vi "CPP_CalcTubingCorrection.vi"() -> (5 "Plug in titles":string[](array[string]), 7 "Plug in values":string[](array[string]))   [LabVIEW 2020]
uses:
  <vilib>/Analysis/baseanly.llb/Mean (DBL).vi
  Globals/Meas_global.vi
  <vilib>/Analysis/NI_AALBase.lvlib
  <vilib>/Analysis/NI_AALPro.lvlib
panel:
  in  "Tab Control":enum32{"TubingCorrection", "Setup"}(tab)
  in  "RefXducer":i32(ring) items=["RV (Ref)", "RV (1)", "RV (2)", "RV (3)", "RV (4)", "RV (5)", "RV (6)", "RV (7)", "RV (8)", "RV (9)", "RV (10)", "RV (11)", "RV (12)", "RV (13)", "RV (14)", "RV (15)", "RV (16)", "RV (17)", "RV (18)", "RV (19)", "RV (20)", "RV (21)", "RV (22)", "RV (23)", "RV (24)", "RV (25)", "RV (26)", "RV (27)", "RV (28)", "RV (29)", "RV (30)", "RV (31)", "RV (32)", "RV (33)", "RV (34)", "RV (35)", "RV (36)", "RV (37)", "RV (38)", "RV (39)", "RV (40)", "RV (41)", "RV (42)", "RV (43)", "RV (44)", "RV (45)", "RV (46)", "RV (47)", "RV (48)", "RV (49)", "RV (50)", "RV (51)", "RV (52)", "RV (53)", "RV (54)", "RV (55)", "RV (56)", "RV (57)", "RV (58)", "RV (59)", "RV (60)", "RV (61)", "RV (62)", "RV (63)", "RV (64)"]
  in  "TestXducer":i32(ring) items=["RV (Ref)", "RV (1)", "RV (2)", "RV (3)", "RV (4)", "RV (5)", "RV (6)", "RV (7)", "RV (8)", "RV (9)", "RV (10)", "RV (11)", "RV (12)", "RV (13)", "RV (14)", "RV (15)", "RV (16)", "RV (17)", "RV (18)", "RV (19)", "RV (20)", "RV (21)", "RV (22)", "RV (23)", "RV (24)", "RV (25)", "RV (26)", "RV (27)", "RV (28)", "RV (29)", "RV (30)", "RV (31)", "RV (32)", "RV (33)", "RV (34)", "RV (35)", "RV (36)", "RV (37)", "RV (38)", "RV (39)", "RV (40)", "RV (41)", "RV (42)", "RV (43)", "RV (44)", "RV (45)", "RV (46)", "RV (47)", "RV (48)", "RV (49)", "RV (50)", "RV (51)", "RV (52)", "RV (53)", "RV (54)", "RV (55)", "RV (56)", "RV (57)", "RV (58)", "RV (59)", "RV (60)", "RV (61)", "RV (62)", "RV (63)", "RV (64)"]
  out "Time Traces":cluster{dbl, dbl, dbl[][]}(graph)
  out "Spectra":cluster{dbl, "df (Hz)":dbl, dbl[][]}(graph)
  in  "stop":bool
  in  "Pause Button":bool
  in  "Pause(ms)":u32=500
  in  "Coherence Threshold":dbl=0.98
  out "Coefficients Smoothed and Normalized":bool
  in  "Decimate Correction File?":bool=TRUE
  in  "Smooth Correction File?":bool=TRUE
  in  "CorrectionFileDestinationPath":path
  in  "fcut (Hz)":dbl=1000.0
  in  "Cutoff type":string(combo)="Brickwall"
  out "SD(boosted)":dbl format="%.3e"
  out "SD(ref)":dbl format="%.3e"
  out "SD(Boostederror%)":dbl format="%#_3g"
  out "Current Block No":i32
  in  "LowFrequencySmoothingFloor":dbl
  in  "LowFrequencySmoothingCeiling":dbl
  in  "ExistingTubingCorrectionFile":path
  in  "Apply Phase Correction?":bool=TRUE
  in  "Save Files?":bool
  in  "Use Existing Correction File?":bool
  out "df (Hz)":dbl format="%.6f"
  in  "Decimation Term":i32=10
  out "OutputString":string
  in  "N Points To Average Either Side":i32=10
  in  "Force Phase 0 Intercept?":bool=TRUE
  out "SD(muted)":dbl format="%.3e"
  out "SD(Mutederror%)":dbl format="%#_3g"
  # "#ToDo Must improve bottom end smoothing- DO NOT clamp to 1.00!!"
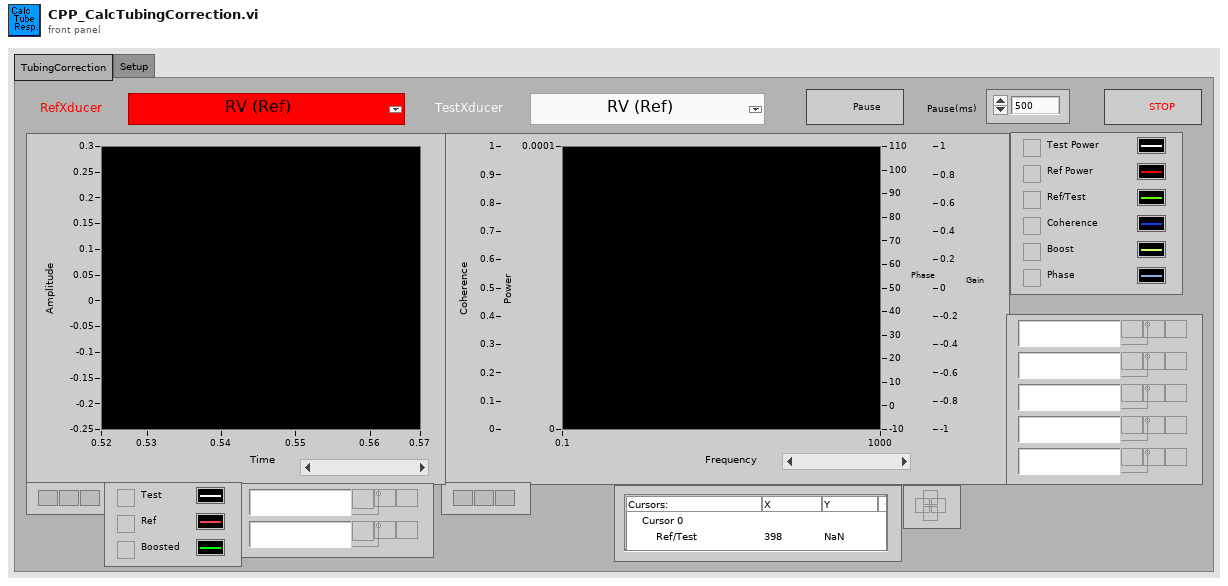
[diagram p1: front panel]
types:
  T1 = typedef "Analysis_info_cluster.ctl" = cluster{"Colour":u32, "Inst type":T2, "Inst name":string, "Symbol":string, "Code name":string, "Extra Info":string, "Inst Array":T3, "Extra Titles":string[], "Extra Values":string[], "U":dbl, "u^2":dbl, "u^3":dbl, "u^4":dbl, "Skew_u":dbl, "Kurt_u":dbl, "Sd Error in Mean":dbl, "% u'/U":dbl, "X":dbl, "Y":dbl, "Z":dbl, "Timescale integral Estimate":dbl, "Sd Error in Variance":dbl, "Calib File":path, "Calib Constants":dbl[], "Output Position":bool, "Stats":enum16{"None", "Basic", "Full"}, "Av Sampling Rate":dbl, "Av No of Samples":dbl, "Total Meas Time (s)":dbl, "ADAM Ch Name":string, "Max value":dbl, "Min value":dbl, "Req Sample Rate Hz":dbl, "Sync Delay Time (s)":dbl, "Ch No":i16, "Device":string, "Use Latest Calib":bool, "Port":string, "Metadata Ch Names":string[], "Metadata Ch Values":string[], "Label":string}
  T2 = typedef "Inst_type.ctl" = enum16{"Raw voltage", "Raw with zero offsetting", "Propeller anemometer", "Pressure Transducer", "Pitot-static tube", "Hot wire", "Cross wire 1", "Cross wire 2", "Generic Linear", "Generic Polynomial", "Generic BackPoly", "Fast FID", "Thermocouple", "Cold wire", "Pulsed Wire", "LDA Vel", "LDA Tran time", "LDA Arr time", "Microphone"}
  T3 = typedef "Instrument_Array.ctl" = enum16{"PWA", "LDA", "Analogue"}
  T4 = typedef "Time_Trace_Cluster.ctl" = cluster{"Weighting":dbl[], "Time (s)":dbl[], "Voltage":dbl[], "Eng Values":dbl[]}
  T5 = enum16{"open", "replace", "create", "open or create", "replace or create", "replace or create with confirmation"}
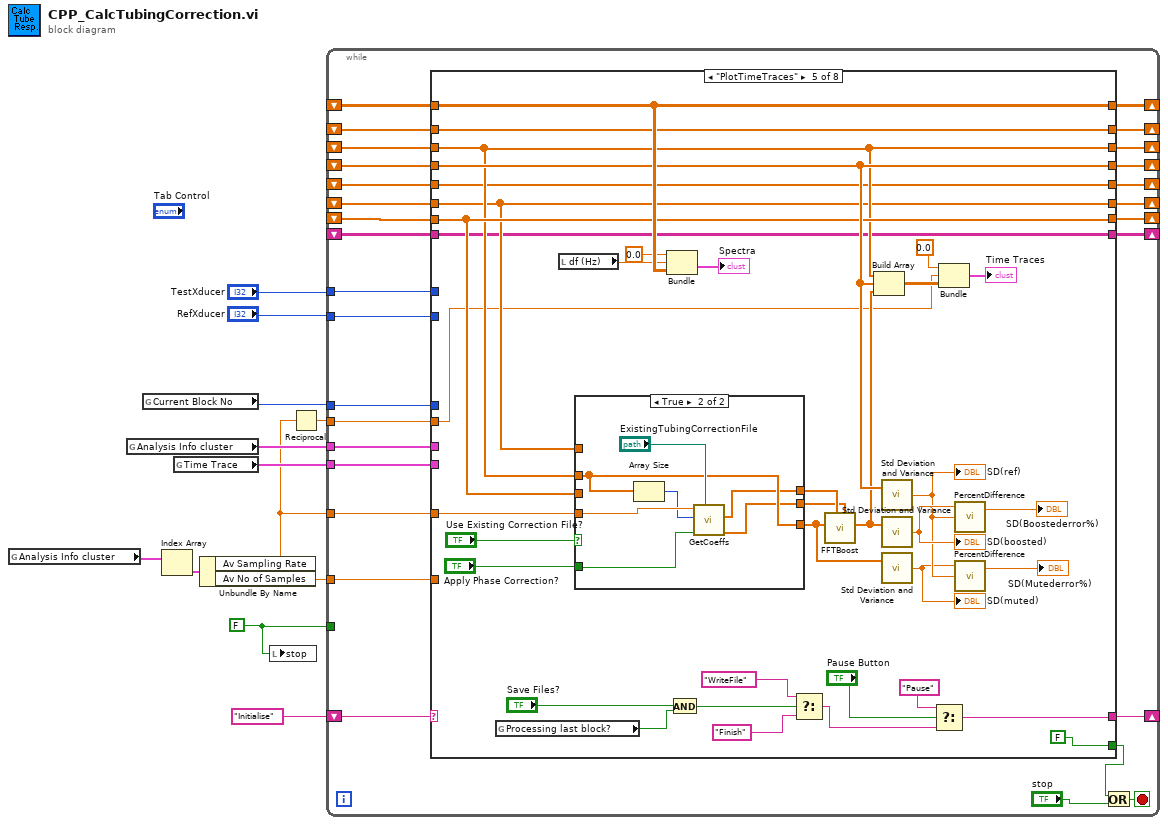
[diagram p0: block diagram]
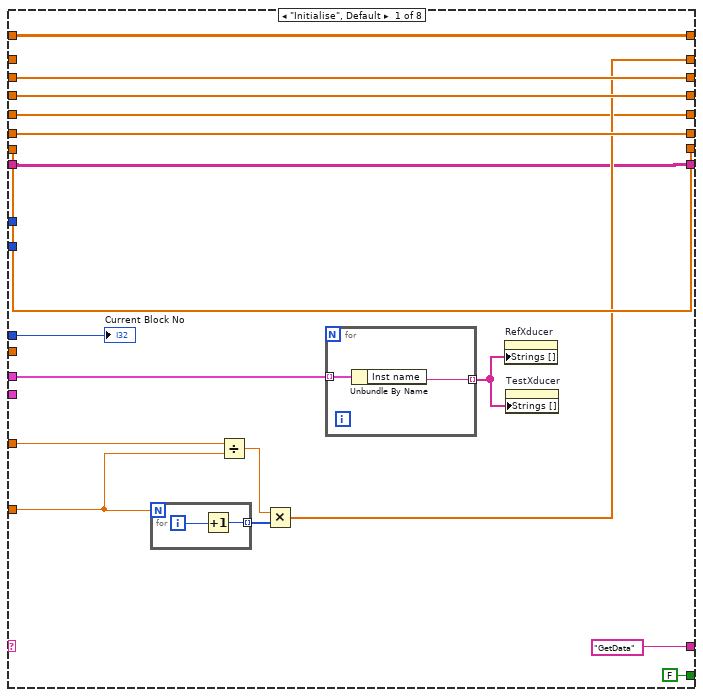
[diagram p2: hidden frame]
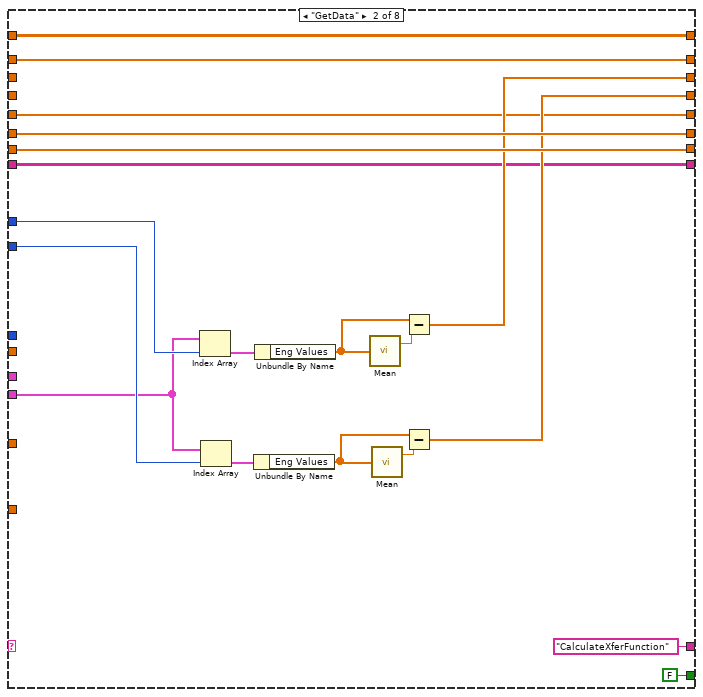
[diagram p3: hidden frame]
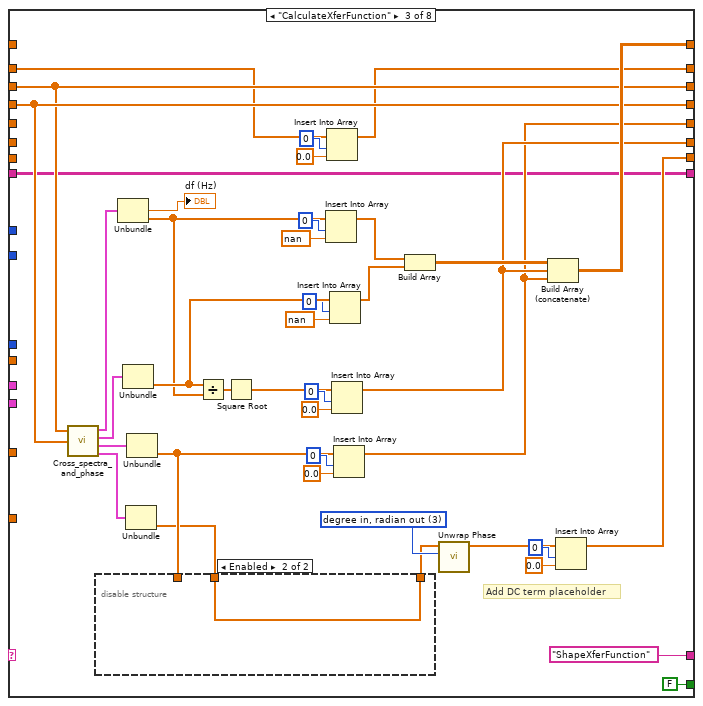
[diagram p4: hidden frame]
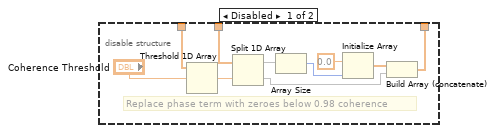
[diagram p5: hidden frame]
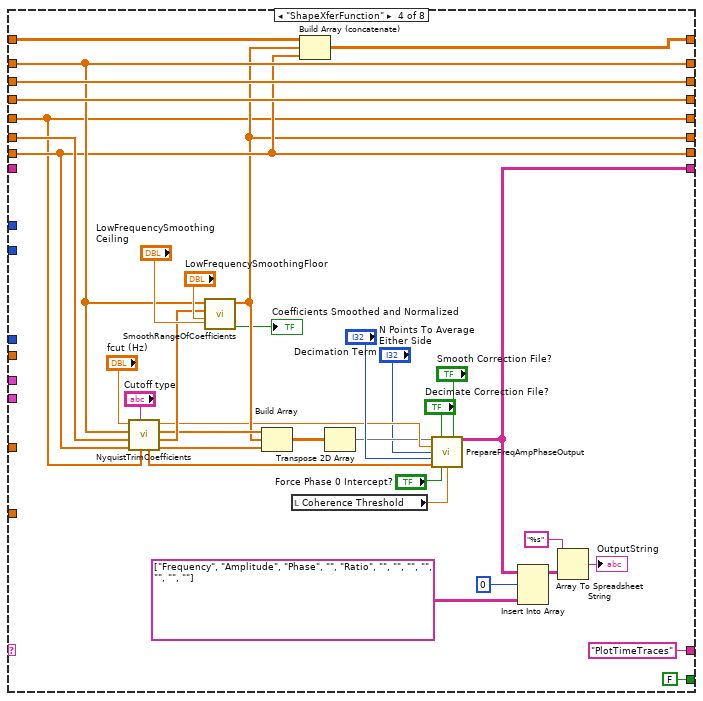
[diagram p6: hidden frame]
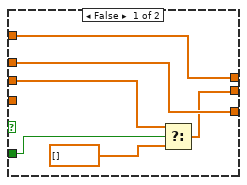
[diagram p7: hidden frame]
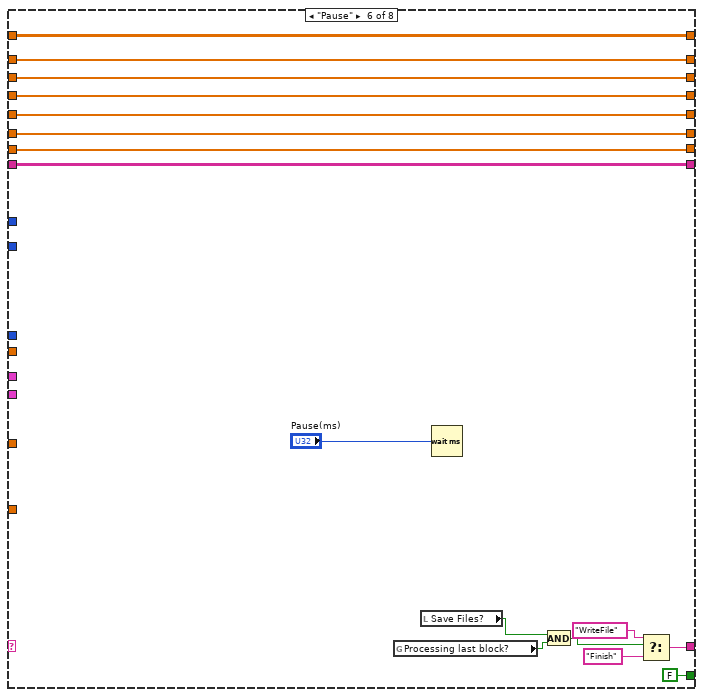
[diagram p8: hidden frame]
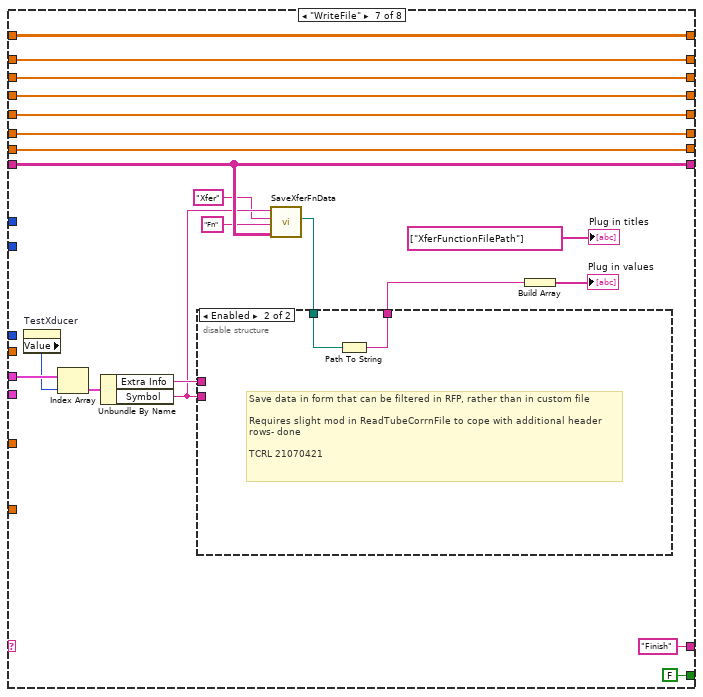
[diagram p9: hidden frame]
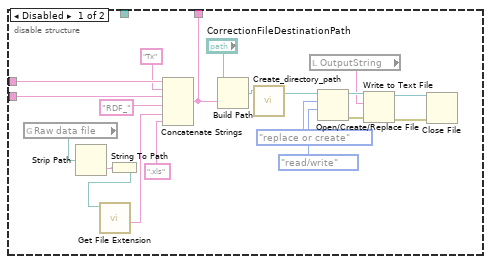
[diagram p10: hidden frame]
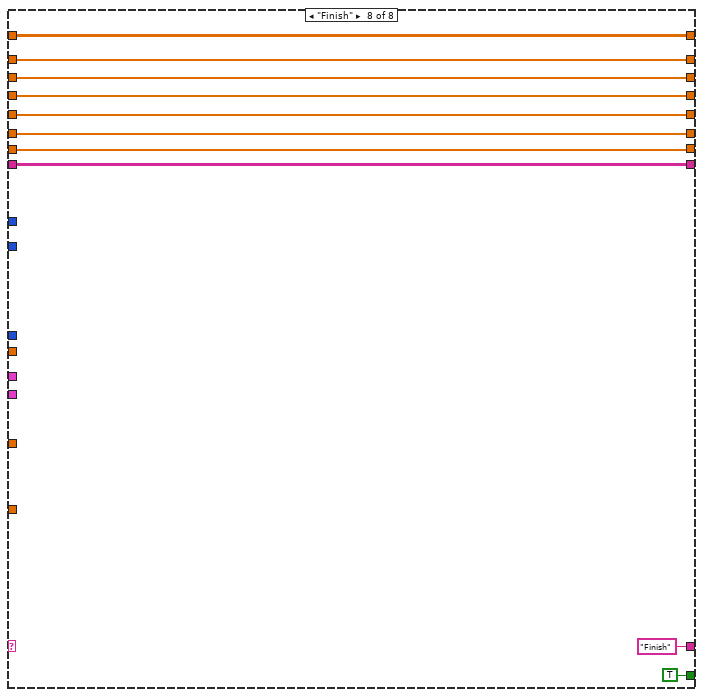
[diagram p11: hidden frame]
diagram:
  w11 = FALSE ("stop")
  n1 = global read "Meas_global.vi" "Analysis Info cluster"() -> (w5:T1[])
  n2 = global read "Meas_global.vi" "Analysis Info cluster"() -> (w8:T1[])
  n3 = global read "Meas_global.vi" "Current Block No"() -> (w9:i32)
  n4 = Index Array(array=w5) -> (element=w3:T1)  [unwired: 1 in]
  n5 = global read "Meas_global.vi" "Time Trace"() -> (w7:T4[])
  n6 = Unbundle By Name(w3) -> ("Av Sampling Rate"=w1:dbl, "Av No of Samples"=w2:dbl)
  n7 = local write "stop"(w11) -> ()
  n8 = Reciprocal(x=w1) -> (1/x=w6:dbl)
  n9 = while {
    shift-right: [w37] -> _
    shift-left: "Initialise" -> [w41]
    tunnel: w8 -> [w40]
    tunnel: "RefXducer" -> [w38]
    tunnel: w6 -> [w36]
    tunnel: w11 -> [_]
    shift-right: [w35] -> _
    shift-left: _ -> [w33]
    shift-right: [w34] -> _
    shift-left: _ -> [w32]
    tunnel: w9 -> [w31]
    tunnel: w7 -> [w30]
    shift-right: [w29] -> _
    shift-left: _ -> [w28]
    tunnel: w1 -> [w27]
    shift-right: [w26] -> _
    shift-left: _ -> [w25]
    tunnel: w2 -> [w24]
    shift-right: [w23] -> _
    shift-left: _ -> [w22]
    shift-right: [w21] -> _
    shift-left: _ -> [w20]
    tunnel: "TestXducer" -> [w39]
    shift-right: [w16] -> _
    shift-left: _ -> [w15]
    shift-right: [w14] -> _
    shift-left: _ -> [w13]
    stop <- w18 stop-if-true
    n10 = case shown="\"PlotTimeTraces\"" w41 {
      tunnel: w40 -> [w54 _ _ _ _ _ w243 _]
      tunnel: w39 -> [_ w81 _ _ _ _ _ _]
      tunnel: w38 -> [_ w80 _ _ _ _ _ _]
      tunnel: ["GetData" "CalculateXferFunction" "ShapeXferFunction" ("t") "PlotTimeTraces" ("t") w201 w223 "Finish" ("t") "Finish" ("t")] -> w37
      tunnel: w36 -> [_ _ _ _ w177 _ _ _]
      tunnel: [w57 w67 w93 w167 w192 w233 w254 w286] -> w35
      tunnel: [w56 w66 w114 w166 w194 w232 w253 w285] -> w34
      tunnel: w33 -> [w57 _ w93 w167 w192 w233 w254 w286]
      tunnel: w32 -> [w56 _ w114 w166 w194 w232 w253 w285]
      tunnel: w31 -> [w55 _ _ _ _ _ _ _]
      tunnel: w30 -> [_ w76 _ _ _ _ _ _]
      tunnel: [w52 w74 w100 w145 w190 w229 w250 w282] -> w26
      tunnel: [w53 w75 w95 w156 w193 w230 w251 w283] -> w29
      tunnel: w28 -> [w53 w75 _ w156 w193 w230 w251 w283]
      tunnel: w27 -> [w51 _ _ _ w176 _ _ _]
      tunnel: w25 -> [w52 w74 _ w157 w190 w229 w250 w282]
      tunnel: w24 -> [w50 _ _ _ _ _ _ _]
      tunnel: [w49 w73 w88 w158 w191 w228 w249 w281] -> w23
      tunnel: w22 -> [_ w73 w89 w158 w191 w228 w249 w281]
      tunnel: [w48 w72 w121 w162 w197 w227 w248 w280] -> w21
      tunnel: w20 -> [w48 w72 _ w163 w197 w227 w248 w280]
      tunnel: [FALSE FALSE FALSE FALSE FALSE FALSE FALSE TRUE] -> w17
      tunnel: [w43 w64 w83 w136 w174 w219 w240 w278] -> w16
      tunnel: w15 -> [w43 w64 _ w136 w174 w219 w240 w278]
      tunnel: [w42 w63 w82 w133 w169 w218 w238 w277] -> w14
      tunnel: w13 -> [w42 w63 w82 _ w169 w218 w238 w277]
      frame "Initialise", Default {
        n11 = for {
          N: w50 -> [_]
          tunnel: [w59] -> w46 mode=indexing
          i -> [w60]
          n12 = Increment(x=w60) -> (x+1=w59:i32)
        }
        n13 = Divide(x=w51, y=w50) -> (x/y=w45:dbl)
        n14 = Multiply(x=w45, y=w46) -> (x*y=w49:dbl[])
        n15 = for {
          tunnel: w54 -> [w62] mode=indexing
          tunnel: [w61] -> w47 mode=indexing
          n16 = Unbundle By Name(w62) -> ("Inst name"=w61:string)
        }
        n17 = property on="RefXducer" class="Ring (strict)"("Strings []"=w47) -> ()  [unwired: 2 in, 2 out]
        n18 = property on="TestXducer" class="Ring (strict)"("Strings []"=w47) -> ()  [unwired: 2 in, 2 out]
        "Current Block No" <- w55
      }
      frame "GetData" {
        n19 = Index Array(array=w76, index=w81) -> (element=w78:T4)
        n20 = Index Array(array=w76, index=w80) -> (element=w77:T4)
        n21 = Unbundle By Name(w77) -> ("Eng Values"=w68:dbl[])
        n22 = Unbundle By Name(w78) -> ("Eng Values"=w69:dbl[])
        n23 = call-poly <vilib>:"Mean.vi"("X"=w69) -> ("mean"=w70:dbl)  [unwired: 1 out]
        n24 = call-poly <vilib>:"Mean.vi"("X"=w68) -> ("mean"=w71:dbl)  [unwired: 1 out]
        n25 = Subtract(x=w69, y=w70) -> (x-y=w67:dbl[])
        n26 = Subtract(x=w68, y=w71) -> (x-y=w66:dbl[])
      }
      frame "CalculateXferFunction" {
        w116 = 3 items=["radian in, radian out", "radian in, degree out", "degree in, degree out", "degree in, radian out"] ("phase unit")
        # "Add DC term placeholder"
        n27 = call "Cross_spectra_and_phase.vi"("U1"=w93, "U2"=w114) -> ("U1 spectra"=w120:cluster{dbl, dbl, dbl[]}, "U2 spectra"=w119:cluster{dbl, dbl, dbl[]}, "U1 U2 coherence"=w118:cluster{dbl, dbl, "Coherence array":dbl[]}, "U1 U2 phase"=w117:cluster{dbl, dbl, "Phase array":dbl[]})  [unwired: 3 out]
        n28 = Unbundle(w120) -> (→"df (Hz)":dbl, w92:dbl[])  [unwired: 1 out]
        n29 = Unbundle(w119) -> (w104:dbl[])  [unwired: 2 out]
        n30 = Unbundle(w117) -> ("Phase array"=w86:dbl[])  [unwired: 2 out]
        n31 = Unbundle(w118) -> ("Coherence array"=w87:dbl[])  [unwired: 2 out]
        n32 = disable-structure shown="Enabled" {
          disable-tunnel: w87 -> [w131 _]
          disable-tunnel: w86 -> [w129 w132]
          disable-tunnel: [w124 w132] -> w85
          frame Disabled {
            # "Replace phase term with zeroes below 0.98 coherence"
            n33 = Threshold 1D Array(2:"Coherence Threshold", 3:w131) -> (0:w130:dbl)  [unwired: 1 in]
            n34 = Split 1D Array(array=w129, index=w130) -> (first subarray=w128:dbl[], second subarray=w127:dbl[])
            n35 = Array Size(array=w128) -> (size(s)=w126:i32)
            n36 = Initialize Array(0.0 ("element"), w126) -> (w125:dbl[])
            n37 = Build Array (concatenate)(w125, w127) -> (w124:dbl[])
          }
          frame Enabled {
          }
        }
        n38 = Divide(x=w104, y=w92) -> (x/y=w112:dbl[])
        n39 = Square Root(x=w112) -> (sqrt(x)=w101:dbl[])
        n40 = Insert Into Array(array=w92, index=0, new element=nan ("new element/subarray")) -> (w106:dbl[])
        n41 = Insert Into Array(array=w89, index=0, new element=0.0 ("new element/subarray")) -> (w88:dbl[])
        n42 = Insert Into Array(array=w104, index=0, new element=nan ("new element/subarray")) -> (w105:dbl[])
        n43 = Insert Into Array(array=w101, index=0, new element=0.0 ("new element/subarray")) -> (w100:dbl[])
        n44 = Insert Into Array(array=w87, index=0, new element=0.0 ("new element/subarray")) -> (w83:dbl[])
        n45 = Build Array(w106, w105) -> (w113:dbl[][])
        n46 = call <vilib>:"Unwrap Phase.vi"("phase unit"=w116, "Phase"=w85) -> ("Unwrapped Phase"=w84:dbl[])  [unwired: 8 in, 1 out]
        n47 = Build Array (concatenate)(w113, w100, w83) -> (w121:dbl[][])
        n48 = Insert Into Array(array=w84, index=0, new element=0.0 ("new element/subarray")) -> (w95:dbl[])
      }
      frame "ShapeXferFunction" {
        n49 = call "NyquistTrimCoefficients.vi"("Coherence"=w136, "Cutoff type"="Cutoff type", "InterpolatedPhase"=w156, "InterpolatedCoefficients"=w157, "Frequencies"=w158, "fcut (Hz)"="fcut (Hz)") -> ("NyquistLimitedPhase"=w149:dbl[], "NyquistLimitedCoefficients"=w148:dbl[], "NyquistLimitedFrequency"=w147:dbl[], "fcut Index"=w144:dbl, "NyquistLimitedCoherence"=w135:dbl[])  [unwired: 1 in]
        n50 = call "SmoothRangeOfCoefficients.vi"("LFSmoothingCeiling"="LowFrequencySmoothingCeiling", "LFSmoothingFloor"="LowFrequencySmoothingFloor", "NyquistLimitedCoefficients In"=w148, "Frequencies In"=w158) -> ("Coefficients Smoothed and Normalized"=→"Coefficients Smoothed and Normalized":bool, "NyquistLimitedCoefficients Out"=w145:dbl[])  [unwired: 5 in, 1 out]
        n51 = Build Array(w147, w145, w149) -> (w141:dbl[][])
        n52 = local read "Coherence Threshold"() -> (w134:dbl)
        n53 = Build Array (concatenate)(w163, w145, w156) -> (w162:dbl[][])
        n54 = Transpose 2D Array(2D array=w141) -> (transposed array=w140:dbl[][])
        n55 = call "PrepareFreqAmpPhaseOutput.vi"("Array in"=w140, "Decimate Correction File?"="Decimate Correction File?", "Smooth Correction File?"="Smooth Correction File?", "fcut Index"=w144, "N Points To Average Either Side"="N Points To Average Either Side", "Decimation Term"="Decimation Term", "Coherence"=w135, "Force Phase 0 Intercept?"="Force Phase 0 Intercept?", "Coherence Threshold"=w134) -> ("Array out"=w133:string[][])  [unwired: 6 in]
        n56 = Insert Into Array(array=w133, index (row)=0, new element=string[][] [["Frequency", "Amplitude", "Phase"], ["", "Ratio", ""], ["", "", ""], ["", "", ""]]) -> (w152:string[][])  [unwired: 1 in]
        n57 = Array To Spreadsheet String(array=w152, 3:"%s" ("format string")) -> (spreadsheet string=→"OutputString":string)  [unwired: 1 in]
      }
      frame "PlotTimeTraces" {
        n58 = global read "Meas_global.vi" "Processing last block?"() -> (w184:bool)
        n59 = local read "df (Hz)"() -> (w180:dbl)
        n60 = case shown="True" "Use Existing Correction File?" {
          tunnel: w193 -> [w207 _]
          tunnel: w192 -> [w210 w214]
          tunnel: w190 -> [w209 _]
          tunnel: w176 -> [_ w216]
          tunnel: [w209 w213] -> w179
          tunnel: [w210 w214] -> w173
          tunnel: "Apply Phase Correction?" -> [w208 w212]
          tunnel: [w205 w211] -> w168
          frame False {
            n61 = Select(t=w207, s=w208, f=dbl[] [] ("NyquistLimitedPhase")) -> (s? t:f=w205:dbl[])
          }
          frame True {
            n62 = Array Size(array=w214) -> (size(s)=w215:i32)
            n63 = call "GetCoeffs.vi"("PathToFile"="ExistingTubingCorrectionFile", "Apply Phase Correction?"=w212, "SignalLength"=w215, "fs (Hz)"=w216) -> ("NyquistLimitedPhase"=w211:dbl[], "NyquistLimitedCoefficients"=w213:dbl[])  [unwired: 6 in]
          }
        }
        n64 = Bundle(0.0, "df (Hz)"=w180, w197) -> (→"Spectra":cluster{dbl, "df (Hz)":dbl, dbl[][]})  [unwired: 1 in]
        n65 = And(x="Save Files?", y=w184) -> (x .and. y?=w183:bool)
        n66 = Select(t="WriteFile", s=w183, f="Finish") -> (s? t:f=w187:string)
        n67 = call "FFTBoost.vi"("PhaseCorrection"=w168, "CompensationCoefficients"=w179, "mutedData"=w173) -> ("boostedData"=w178:dbl[])  [unwired: 1 in, 7 out]
        n68 = Build Array(w192, w194, w178) -> (w200:dbl[][])
        n69 = call <vilib>:"Std Deviation and Variance.vi"("X"=w194) -> ("standard deviation"=w172:dbl)  [unwired: 1 in, 2 out]
        "SD(ref)" <- w172
        n70 = call <vilib>:"Std Deviation and Variance.vi"("X"=w178) -> ("standard deviation"=w195:dbl)  [unwired: 1 in, 2 out]
        "SD(boosted)" <- w195
        n71 = call <vilib>:"Std Deviation and Variance.vi"("X"=w173) -> ("standard deviation"=w171:dbl)  [unwired: 1 in, 2 out]
        "SD(muted)" <- w171
        n72 = Select(t="Pause", s="Pause Button", f=w187) -> (s? t:f=w201:string)
        n73 = Bundle(0.0, w177, w200) -> (→"Time Traces":cluster{dbl, dbl, dbl[][]})  [unwired: 1 in]
        n74 = call "PercentDifference.vi"("Basis"=w172, "Comparee"=w195) -> ("PercentageDifference"=→"SD(Boostederror%)":dbl)  [unwired: 1 in, 1 out]
        n75 = call "PercentDifference.vi"("Basis"=w172, "Comparee"=w171) -> ("PercentageDifference"=→"SD(Mutederror%)":dbl)  [unwired: 1 in, 1 out]
      }
      frame "Pause" {
        n76 = global read "Meas_global.vi" "Processing last block?"() -> (w221:bool)
        n77 = local read "Save Files?"() -> (w222:bool)
        n78 = Wait (ms)(milliseconds to wait="Pause(ms)") -> ()  [unwired: 1 out]
        n79 = And(x=w222, y=w221) -> (x .and. y?=w220:bool)
        n80 = Select(t="WriteFile", s=w220, f="Finish") -> (s? t:f=w223:string)
      }
      frame "WriteFile" {
        n81 = property on="TestXducer" class="Ring (strict)"() -> ("Value"=w241:i32)  [unwired: 2 in, 2 out]
        n82 = Index Array(array=w243, index=w241) -> (element=w242:T1)
        n83 = Unbundle By Name(w242) -> ("Extra Info"=w239:string, "Symbol"=w237:string)
        n84 = call "SaveXferFnData.vi"("XferFn"=w238, "ColumnTitle2"="Fn", "ColumnTile1"="Xfer", "Inst (file) name"=w237) -> ("Path name Out"=w234:path)  [unwired: 3 in]
        n85 = disable-structure shown="Enabled" {
          disable-tunnel: [w274 w275] -> w244
          disable-tunnel: w239 -> [w259 _]
          disable-tunnel: w237 -> [w255 _]
          disable-tunnel: w234 -> [_ w276]
          frame Disabled {
            n86 = global read "Meas_global.vi" "Raw data file"() -> (w263:path)
            n87 = Strip Path(path=w263) -> (name=w262:string)  [unwired: 1 out]
            n88 = String To Path(string=w262) -> (path=w261:path)
            n89 = call <vilib>:"Get File Extension.vi"("file"=w261) -> ("filename without extension"=w256:string)  [unwired: 6 in, 4 out]
            n90 = Concatenate Strings(w259, "Tx" ("string"), w255, "RDF_" ("string"), w256, ".xls" ("string")) -> (w274:string)
            n91 = Build Path(base path="CorrectionFileDestinationPath", name or relative path=w274) -> (appended path=w266:path)
            n92 = call "Create_directory_path.vi"("Path name"=w266) -> ("Path name Out"=w265:path)  [unwired: 2 in, 1 out]
            n93 = local read "OutputString"() -> (w269:string)
            n94 = Open/Create/Replace File(file path (use dialog)=w265, operation (0:open)=T5."replace or create", access (0:read/write)=enum16{"read/write", "read-only", "write-only"}."read/write") -> (refnum out=w270:refnum<file>, error out=w271:errorcluster)  [unwired: 3 in, 1 out]
            n95 = Write to Text File(file (use dialog)=w270, text=w269, error in=w271) -> (refnum out=w267:refnum<file>, error out=w268:errorcluster)  [unwired: 1 in, 1 out]
            n96 = Close File(refnum=w267, error in=w268) -> ()  [unwired: 2 out]
          }
          frame Enabled {
            # "Save data in form that can be filtered in RFP, rather than in custom file\n\nRequires slight mod in ReadTubeCorrnFile to cope with additional header rows- done\n\nTCRL 21070421"
            n97 = Path To String(path=w276) -> (string=w275:string)
          }
        }
        n98 = Build Array(w244) -> (→"Plug in values":string[])
        "Plug in titles" <- string[] ["XferFunctionFilePath"] ("Add in values")
      }
      frame "Finish" {
      }
    }
    n99 = Or(x=w17, y="stop") -> (x .or. y?=w18:bool)
  }
